vi "VI Tree.vi"   [LabVIEW 2011, in "Hokuyo URG Series.lvlib"]
doc: "This is the instrument driver for the Hokuyo URG Series. The VI Tree displays all the user-callable VIs of the instrument driver in an organized table."
uses:
  Hokuyo URG Series.lvlib
  Initialize-Standard.vi
panel:
  # "(c) 2009 National Instruments.  ALL RIGHTS RESERVED."
  # "SEE DIAGRAM\nFOR VI TREE."
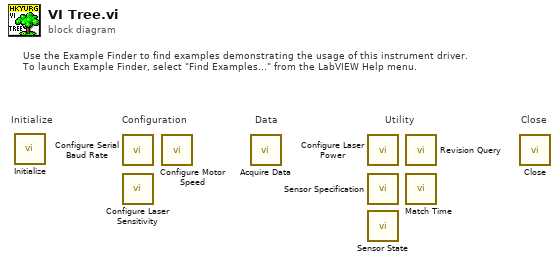
[diagram p0: block diagram]
diagram:
  # "Use the Example Finder to find examples demonstrating the usage of this instrument driver.\nTo launch Example Finder, select \"Find Examples...\" from the LabVIEW Help menu."
  # "Configuration"
  # "Utility"
  # "Data"
  # "Close"
  # "Initialize"
  n1 = call-poly "Initialize.vi"() -> ()  [unwired: 10 in, 2 out]
  n2 = call "Configure Serial Baud Rate.vi"() -> ()  [unwired: 10 in, 2 out]
  n3 = call "Configure Laser Sensitivity.vi"() -> ()  [unwired: 10 in, 2 out]
  n4 = call "Configure Motor Speed.vi"() -> ()  [unwired: 10 in, 2 out]
  n5 = call "Acquire Data.vi"() -> ()  [unwired: 8 in, 4 out]
  n6 = call "Configure Laser Power.vi"() -> ()  [unwired: 10 in, 2 out]
  n7 = call "Sensor Specification.vi"() -> ()  [unwired: 9 in, 3 out]
  n8 = call "Sensor State.vi"() -> ()  [unwired: 9 in, 3 out]
  n9 = call "Revision Query.vi"() -> ()  [unwired: 8 in, 4 out]
  n10 = call "Match Time.vi"() -> ()  [unwired: 9 in, 3 out]
  n11 = call "Close.vi"() -> ()  [unwired: 11 in, 1 out]
